vi "Get All LV Class Files From Search Paths.vi"(11 "error in (no error)":errorcluster) -> (4 "All Files in Dir":path[](array[path]), 15 "error out":errorcluster)   [LabVIEW 2023, in "RFFixtureCharact.Instruments.lvlib" / "Power Meter Factory.lvclass"]
uses:
  Power Meter Factory.lvclass
  Common/RFCalAndFixtureCharact.Common.lvlib
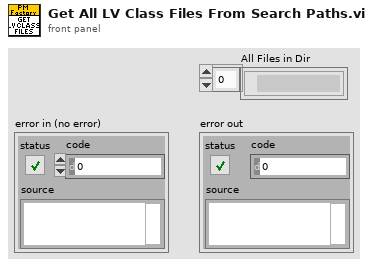
[diagram p1: front panel]
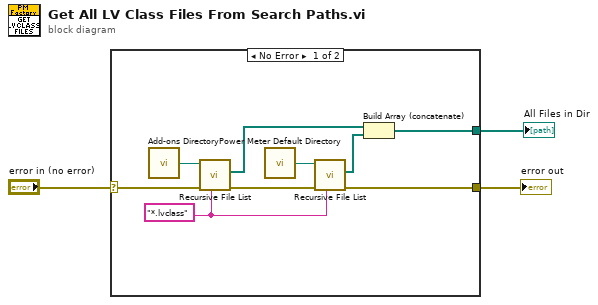
[diagram p0: block diagram]
diagram:
  n1 = case shown="No Error" "error in (no error)" {
    selector: "error in (no error)" -> [w6 w13]
    tunnel: [w10 _] -> w3
    tunnel: [w5 w13] -> w1
    frame No Error {
      w4 = "*.lvclass" ("pattern")
      n2 = call "Add-ons Directory.vi"() -> ("path out"=w12:path)  [unwired: 1 in]
      n3 = call <vilib>:"Recursive File List.vi"("pattern"=w4, "error in (no error)"=w6, "Folder Path"=w12) -> ("error out"=w7:errorcluster, "All Files in Dir"=w8:path[])  [unwired: 4 in, 3 out]
      n4 = call "Power Meter Default Directory.vi"() -> ("Path out"=w11:path)  [unwired: 1 in]
      n5 = call <vilib>:"Recursive File List.vi"("pattern"=w4, "error in (no error)"=w7, "Folder Path"=w11) -> ("error out"=w5:errorcluster, "All Files in Dir"=w9:path[])  [unwired: 4 in, 3 out]
      n6 = Build Array (concatenate)(w8, w9) -> (w10:path[])
    }
    frame Error {
    }
  }
  "All Files in Dir" <- w3
  "error out" <- w1
